vi "Auth Extra.vi"(8 "error in (no error)":errorcluster, 10 "authextra in":string="{}", 11 "SecretBasedAuthenticatorBase in":refnum<class "SecretBasedAuthenticatorBase.lvclass">) -> (0 "error out":errorcluster, 2 "authextra":string caption="authextra out", 3 "SecretBasedAuthenticatorBase out":refnum<class "SecretBasedAuthenticatorBase.lvclass">)   [LabVIEW 2020, in "wamplv.lvlib" / "SecretBasedAuthenticatorBase.lvclass"]
uses:
  SecretBasedAuthenticatorBase.lvclass
  SecretBasedAuthenticatorBase.lvclass/SecretBasedAuthenticatorBase.ctl
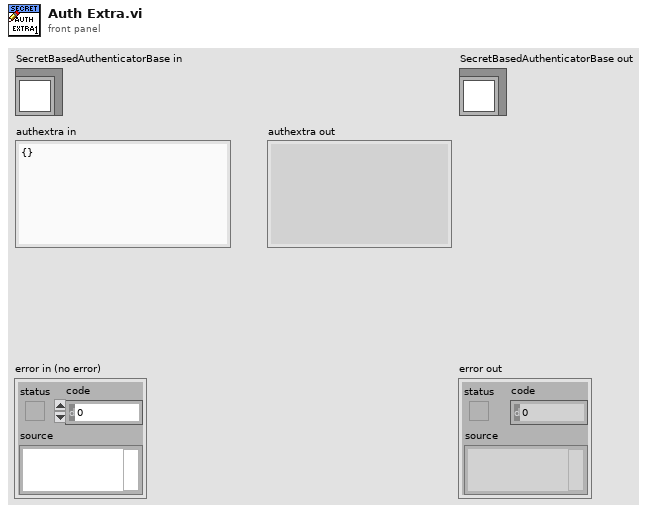
[diagram p1: front panel]
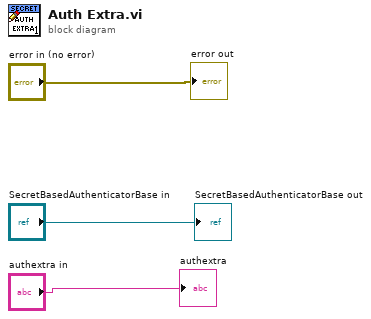
[diagram p0: block diagram]
diagram:
  "error out" <- "error in (no error)"
  "SecretBasedAuthenticatorBase out" <- "SecretBasedAuthenticatorBase in"
  "authextra" <- "authextra in"
